vi "Excel - Get Workbook Reference.vi"(8 "error in (no error)":errorcluster, 11 "Document API in":refnum<class "Document API.lvclass">) -> (0 "error out":errorcluster, 2 "Workbook Reference":refnum<k24>, 3 "Document API out":refnum<class "Document API.lvclass">)   [LabVIEW 2017, in "Document API.lvlib" / "Document API.lvclass"]
uses:
  Document API.lvclass
  C:/Users/Neo/Desktop/Dev_Tools_BR/LabVIEW_NPOI/src/lib/NPOI 2.1.1/NPOI.dll
  lib/NPOI 2.1.1/NPOI.dll
  Document API.lvclass/Document API.ctl
  Get Document Type.vi
  NPOI_Document/npoiDocument/npoiDocument.lvclass
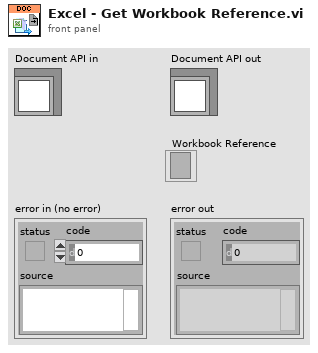
[diagram p1: front panel]
types:
  T1 = typedef "Document API.lvlib/Document API.lvclass/Document Type.ctl" = enum16{"Word", "Excel", "Undefined"}
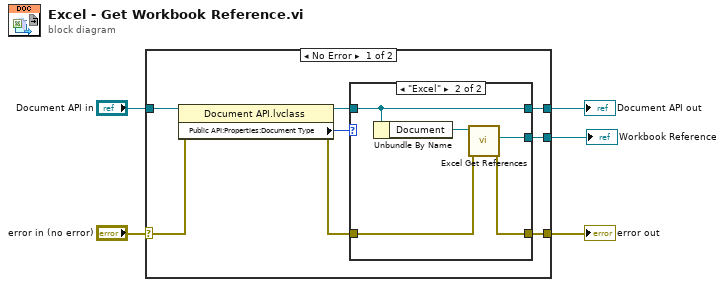
[diagram p0: block diagram]
diagram:
  n1 = case shown="No Error" "error in (no error)" {
    selector: "error in (no error)" -> [w7 w22]
    tunnel: [w11 w22] -> w4
    tunnel: [w9 w21] -> w2
    tunnel: "Document API in" -> [w13 w21]
    tunnel: [w12 _] -> w1
    frame No Error {
      n2 = property class="Document API.lvclass"(reference=w13, error in=w7) -> (reference out=w10:refnum<class "Document API.lvclass">, error out=w6:errorcluster, "Public API:Properties:Document Type"=w8:T1)
      n3 = case shown="\"Excel\"" w8 {
        tunnel: [_ w19] -> w12
        tunnel: w6 -> [w14 w18]
        tunnel: [w14 w17] -> w11
        tunnel: w10 -> [w15 w16]
        tunnel: [w15 w16] -> w9
        frame "Word", Default {
        }
        frame "Excel" {
          n4 = Unbundle By Name(w16) -> ("Document"=w20:refnum<class "npoiDocument.lvclass">)
          n5 = call "Excel Get References.vi"("error in (no error)"=w18, "npoiDocument in"=w20) -> ("error out"=w17:errorcluster, "Workbook.Ref"=w19:refnum<k24>)  [unwired: 6 in, 2 out]
        }
      }
    }
    frame Error {
    }
  }
  "error out" <- w4
  "Document API out" <- w2
  "Workbook Reference" <- w1
